vi "MCU控制.vi"(7 "Enum":enum16{"read", "write", "release", "initial"}(ring), 8 "error in":errorcluster, 10 "write buffer":string, 11 "VISA name":refnum<visa-resource-name>) -> (0 "error out":errorcluster, 2 "read buffer":string)   [LabVIEW 2016]
uses:
  <vilib>/Instr/_visa.llb/VISA Configure Serial Port (Instr).vi
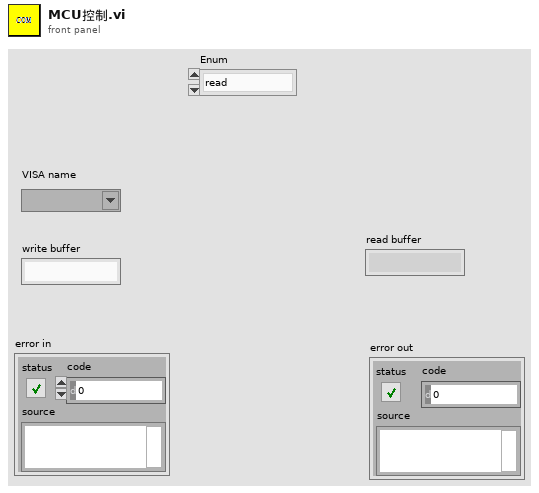
[diagram p1: front panel]
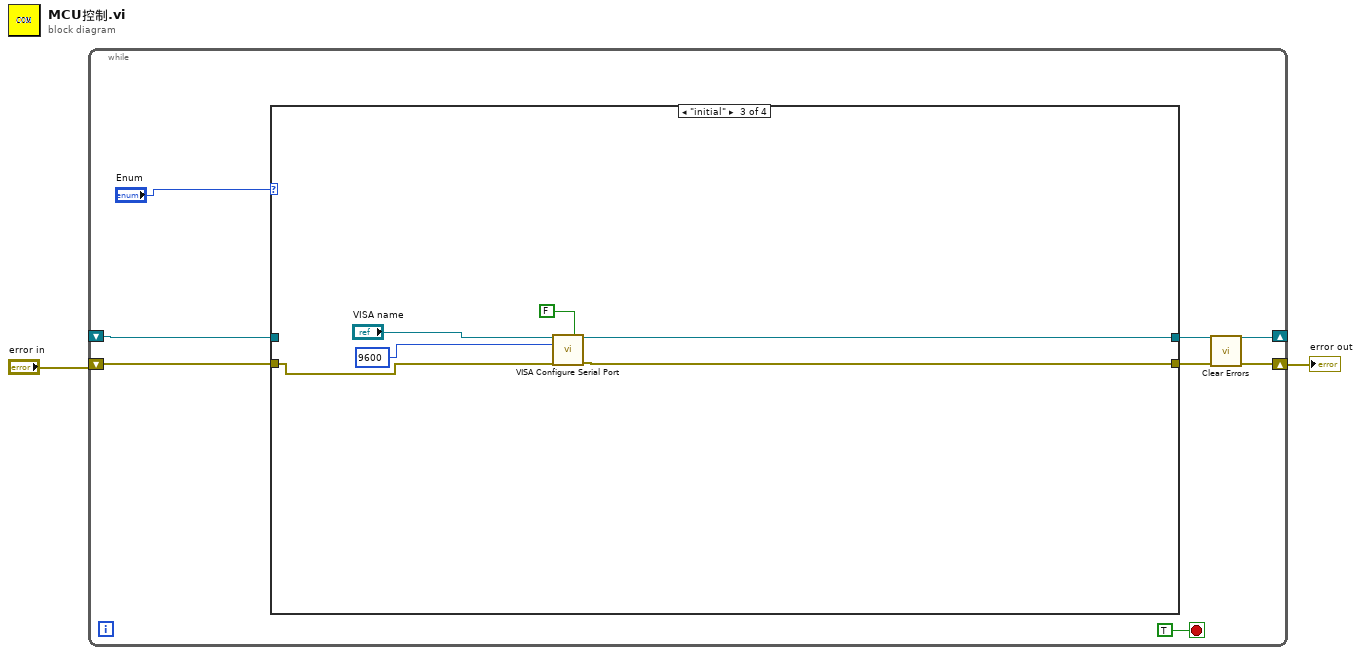
[diagram p0: block diagram]
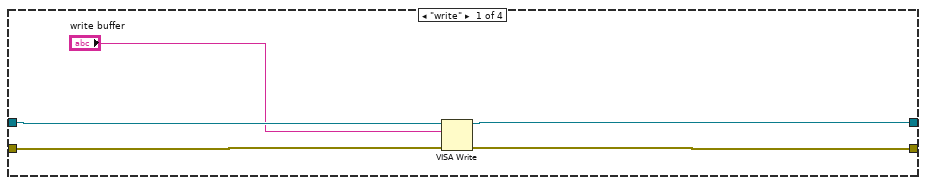
[diagram p2: hidden frame]
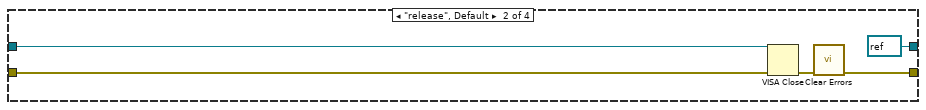
[diagram p3: hidden frame]
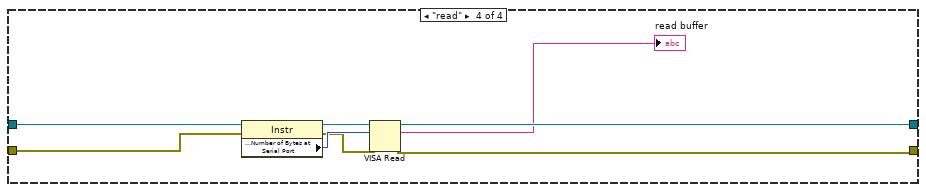
[diagram p4: hidden frame]
diagram:
  n1 = while {
    shift-right: [w9] -> _
    shift-left: _ -> [w8]
    shift-right: [w3] -> w2
    shift-left: "error in" -> [w7]
    stop <- TRUE stop-if-true
    n2 = case shown="\"initial\"" "Enum" {
      tunnel: [w11 refnum<visa-resource-name> refnum ("VISA resource name") w22 w33] -> w9
      tunnel: w8 -> [w14 w18 _ w30]
      tunnel: w7 -> [w13 w16 w20 w26]
      tunnel: [w12 w15 w23 w32] -> w4
      frame "write" {
        n3 = VISA Write(VISA resource name=w14, write buffer="write buffer", error in (no error)=w13) -> (VISA resource name out=w11:refnum<visa-resource-name>, error out=w12:errorcluster)  [unwired: 1 out]
      }
      frame "release", Default {
        n4 = VISA Close(VISA resource name=w18, error in (no error)=w16) -> (error out=w17:errorcluster)
        n5 = call <vilib>:"Clear Errors.vi"("error in (no error)"=w17) -> ("error out"=w15:errorcluster)  [unwired: 5 in, 1 out]
      }
      frame "initial" {
        n6 = call-poly "VISA Configure Serial Port"("VISA resource name"="VISA name", "Enable Termination\nChar (T)"=FALSE ("Enable Termination\nChar (T)"), "baud rate (9600)"=u32 9600, "error in (no error)"=w20) -> ("VISA resource name out"=w22:refnum<visa-resource-name>, "error out"=w23:errorcluster)  [unwired: 10 in]
      }
      frame "read" {
        n7 = property class="Instr"(reference=w30, error in=w26) -> (reference out=w28:refnum<visa-resource-name>, error out=w27:errorcluster, "Serial Settings:Number of Bytes at Serial Port"=w29:u32)
        n8 = VISA Read(VISA resource name=w28, byte count=w29, error in (no error)=w27) -> (VISA resource name out=w33:refnum<visa-resource-name>, read buffer=→"read buffer":string, error out=w32:errorcluster)  [unwired: 1 out]
      }
    }
    n9 = call <vilib>:"Clear Errors.vi"("error in (no error)"=w4) -> ("error out"=w3:errorcluster)  [unwired: 5 in, 1 out]
  }
  "error out" <- w2
